vi "Refname to String (Notifier).vi"(1 "Refname (Notifier)":T1) -> (0 "Refnum Name":string)   [LabVIEW 2015, in "Sprocket.lvlib"]
uses:
  lib/Sprocket.lvlib
  Notifiers.ctl
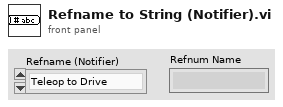
[diagram p1: front panel]
types:
  T1 = typedef "Sprocket.lvlib/Notifiers.ctl" = enum16{"Teleop to Drive", "Teleop to Elevator"}
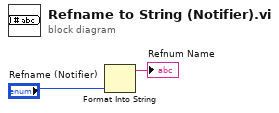
[diagram p0: block diagram]
diagram:
  n1 = Format Into String("Refname (Notifier)") -> (resulting string=→"Refnum Name":string)  [unwired: 3 in, 1 out]
